vi "STScalc.vi"() -> ()   [LabVIEW 2014]
panel:
  in  "preDelay (ms)":dbl=769.1
  in  "number Grids":dbl=24.00933333333333
  out "Size Y":dbl
  in  "ratio":dbl=40.0
  in  "size X":dbl=40.0
  out "ETA":timestamp format="%<%H:%M\n%d/%m/%Y>T"
  in  "Imaging time":dbl=315.0 format="%<%H:%M:%S>t"
  in  "pixel/drift Corr":dbl=160.0
  out "drift corr. every":dbl=52.00884150305552
  in  "QUIT":bool
  in  "# STS       total time":bool=TRUE
  in  "Total time (h)":dbl=24.00933333333333
  in  "#spectra":dbl=15.0
  in  "pts y":dbl=40.0
  in  "pts x":dbl=160.0
  in  "time  STS ms":dbl=769.1
  # "min"
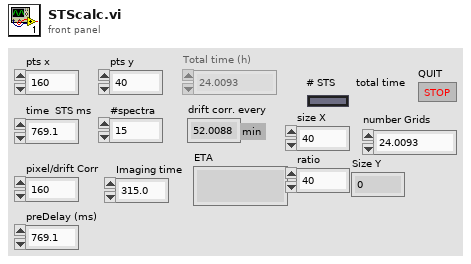
[diagram p1: front panel]
types:
  T1 = enum8{"Enabled", "Disabled", "Disabled and Grayed Out"}
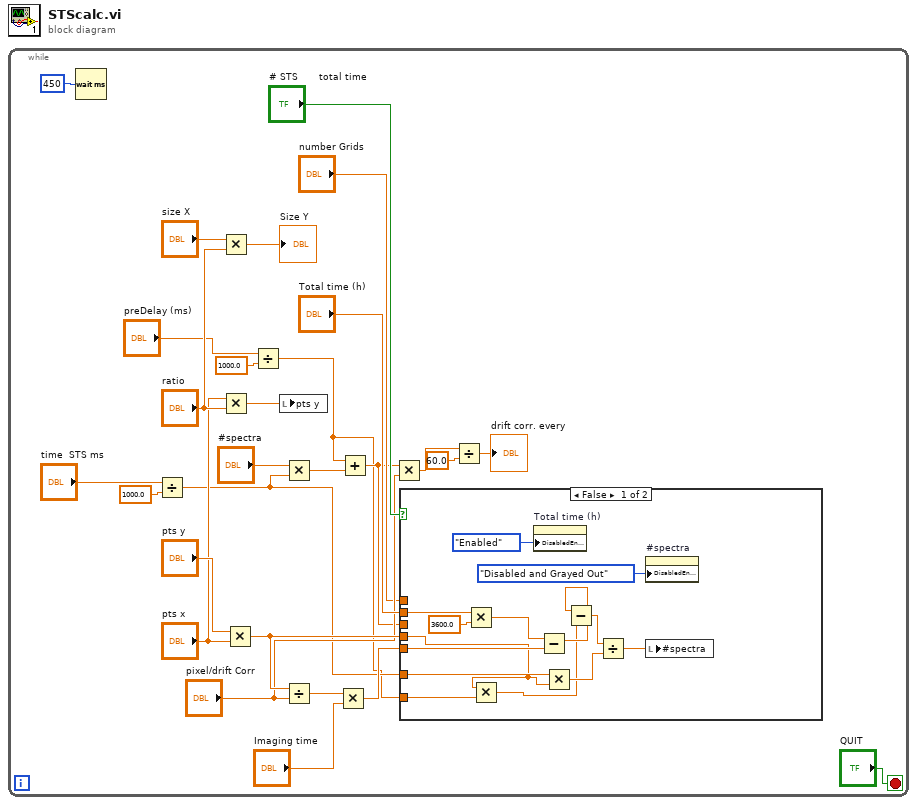
[diagram p0: block diagram]
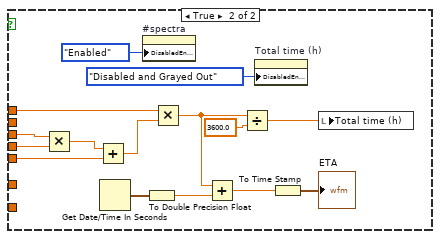
[diagram p2: hidden frame]
diagram:
  n1 = while {
    stop <- "QUIT" stop-if-true
    n2 = Wait (ms)(milliseconds to wait=u32 450) -> ()  [unwired: 1 out]
    n3 = Divide(x="time  STS ms", y=1000.0) -> (x/y=w2:dbl)
    n4 = Multiply(x="size X", y="ratio") -> (x*y=→"Size Y":dbl)
    n5 = Multiply(x="pts x", y="ratio") -> (x*y=w11:dbl)
    n6 = Multiply(x="pts y", y="pts x") -> (x*y=w22:dbl)
    n7 = Divide(x="preDelay (ms)", y=1000.0) -> (x/y=w1:dbl)
    n8 = local write "pts y"(w11) -> ()
    n9 = Multiply(x="#spectra", y=w2) -> (x*y=w3:dbl)
    n10 = Divide(x=w22, y="pixel/drift Corr") -> (x/y=w21:dbl)
    n11 = Multiply(x=w21, y="Imaging time") -> (x*y=w19:dbl)
    n12 = Add(x=w1, y=w3) -> (x+y=w6:dbl)
    n13 = Multiply(x=w6, y="pixel/drift Corr") -> (x*y=w16:dbl)
    n14 = case shown="False" "# STS       total time" {
      tunnel: w22 -> [w30 w57]
      tunnel: "Total time (h)" -> [w42 _]
      tunnel: w19 -> [w35 w52]
      tunnel: "number Grids" -> [_ w45]
      tunnel: w6 -> [_ w43]
      tunnel: w2 -> [w34 _]
      tunnel: w1 -> [w29 _]
      frame False {
        n15 = Multiply(x=w42, y=3600.0) -> (x*y=w36:dbl)
        n16 = Multiply(x=w30, y=w29) -> (x*y=w31:dbl)
        n17 = property on="Total time (h)" class="DigNum (strict)"("DisabledEnum"=T1."Enabled" ("Disabled")) -> ()  [unwired: 2 in, 2 out]
        n18 = Subtract(x=w36, y=w35) -> (x-y=w33:dbl)
        n19 = Multiply(x=w34, y=w30) -> (x*y=w40:dbl)
        n20 = Subtract(x=w33, y=w31) -> (x-y=w32:dbl)
        n21 = Divide(x=w32, y=w40) -> (x/y=w39:dbl)
        n22 = property on="#spectra" class="DigNum (strict)"("DisabledEnum"=T1."Disabled and Grayed Out" ("Disabled")) -> ()  [unwired: 2 in, 2 out]
        n23 = local write "#spectra"(w39) -> ()
      }
      frame True {
        n24 = Multiply(x=w43, y=w57) -> (x*y=w44:dbl)
        n25 = Add(x=w44, y=w52) -> (x+y=w49:dbl)
        n26 = Get Date/Time In Seconds() -> (seconds since 1Jan1904=w51:timestamp)
        n27 = property on="#spectra" class="DigNum (strict)"("DisabledEnum"=T1."Enabled" ("Disabled")) -> ()  [unwired: 2 in, 2 out]
        n28 = To Double Precision Float(number=w51) -> (double precision float=w50:dbl)
        n29 = Multiply(x=w45, y=w49) -> (x*y=w46:dbl)
        n30 = Add(x=w46, y=w50) -> (x+y=w48:dbl)
        n31 = Divide(x=w46, y=3600.0) -> (x/y=w55:dbl)
        n32 = property on="Total time (h)" class="DigNum (strict)"("DisabledEnum"=T1."Disabled and Grayed Out" ("Disabled")) -> ()  [unwired: 2 in, 2 out]
        n33 = To Time Stamp(1:w48) -> (0:→"ETA":timestamp)
        n34 = local write "Total time (h)"(w55) -> ()
      }
    }
    n35 = Divide(x=w16, y=60.0) -> (x/y=→"drift corr. every":dbl)
  }
